vi "MultiChannelType_2D-Array-DBL.vi"(9 "error in":errorcluster, 11 "Array in":dbl[][](array[numeric])) -> (1 "error out":errorcluster, 2 "MultiChannelType":cdb, 3 "Array out":dbl[][](array[numeric]))   [LabVIEW 2020, in "OpenLvVision_OpenCv.lvlib"]
uses:
  OpenLvVision_OpenCv.lvlib
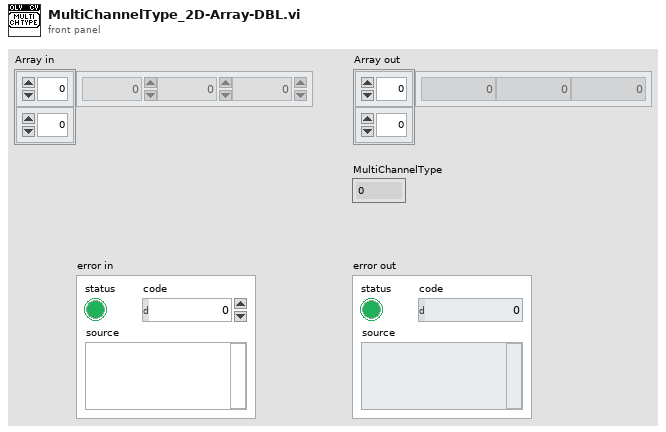
[diagram p1: front panel]
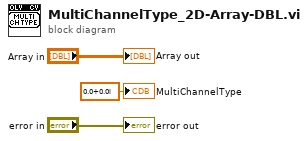
[diagram p0: block diagram]
diagram:
  "error out" <- "error in"
  "Array out" <- "Array in"
  "MultiChannelType" <- cdb 0.0+0.0i
